vi "Start.vi"(8 "error in":errorcluster, 11 "Monitor Execution Unit Implementation in":refnum<class "Monitor Execution Unit.lvclass">) -> (0 "error out":errorcluster, 3 "Monitor Execution Unit Implementation out":refnum<class "Monitor Execution Unit.lvclass">)   [LabVIEW 2020, in "AIM ARINC 664 Engine.lvlib" / "Implementation.lvlib" / "Monitor Execution Unit.lvclass"]
uses:
  Monitor Execution Unit.lvclass
  Monitor Execution Unit.lvclass/Monitor Execution Unit.ctl
  <instrlib>/AIM GmbH/_AIM 664/AIM664LV.lvlib
  <vilib>/Utility/SystemLogging/NI_SystemLogging.lvlib
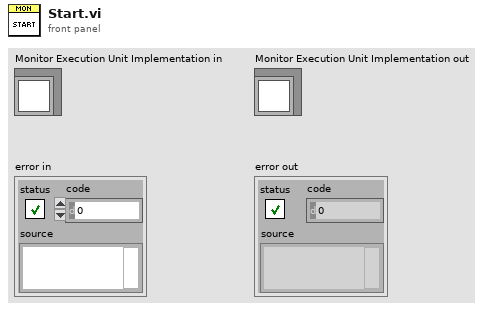
[diagram p1: front panel]
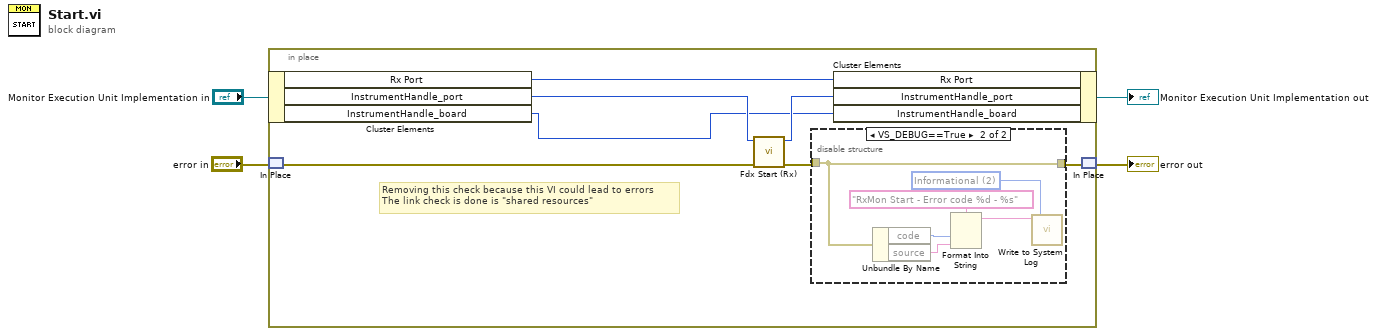
[diagram p0: block diagram]
diagram:
  n1 = in-place {
    # "Removing this check because this VI could lead to errors\nThe link check is done is \"shared resources\""
    n2 = in-place-cluster #1("Monitor Execution Unit Implementation in") -> ("Rx Port"=w7:u32, "InstrumentHandle_port"=w10:u32, "InstrumentHandle_board"=w9:u32)
    n3 = in-place-match #2("error in") -> (w8:errorcluster)
    n4 = call <instrlib>:"Fdx Start (Rx).vi"("error in"=w8, "InstrumentHandle_port in"=w10) -> ("error out"=w6:errorcluster, "InstrumentHandle_port out"=w11:u32)  [unwired: 8 in]
    n5 = disable-structure shown="VS_DEBUG==True" {
      disable-tunnel: w6 -> [w12 w13]
      disable-tunnel: [w12 w13] -> w5
      frame condition #0 (active) {
      }
      frame condition #1 {
        w16 = 2 items=["Error", "Warning", "Informational"] ("severity")
        n6 = Unbundle By Name(w13) -> ("code"=w15:i32, "source"=w14:string)
        n7 = Format Into String(format string="RxMon Start - Error code %d - %s", w15, w14) -> (resulting string=w17:string)  [unwired: 2 in, 1 out]
        n8 = call <vilib>:"Write to System Log.vi"("severity"=w16, "message"=w17) -> ()  [unwired: 9 in, 1 out]
      }
    }
    n9 = in-place-cluster #1("Rx Port"=w7, "InstrumentHandle_port"=w11, "InstrumentHandle_board"=w9) -> (→"Monitor Execution Unit Implementation out":refnum<class "Monitor Execution Unit.lvclass">)
    n10 = in-place-match #2(w5) -> (→"error out":errorcluster)
  }
